vi "User Update Table for Spartan 5.0.vi"(8 "error in (no error)":errorcluster, 11 "Connection Refnum":T1) -> (0 "error out":errorcluster, 3 "Connection Refnum":T1)   [LabVIEW 2011]
uses:
  SI.LIB/ODBC/SQL Controls/Connection Refnum.ctl
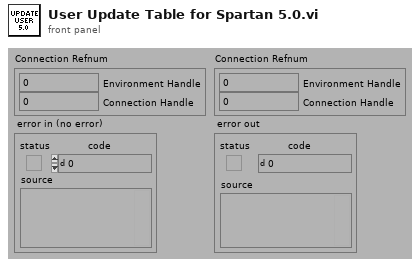
[diagram p1: front panel]
types:
  T1 = typedef "Connection Refnum.ctl" = cluster{"Environment Handle":i32, "Connection Handle":i32}
  T2 = typedef "Statement Refnum.ctl" = cluster{"Statement Handle":i32, "Parameter Number":u16}
  T3 = typedef "User Record.ctl" = cluster{"ixUser":i32, "sxUsername":string, "sLastName":string, "sFirstName":string, "sEmail":string, "sPassword":string, "tLoginTime":timestamp, "sLoginComputer":string, "fAdministrator":bool, "fRunSequences":bool, "fModifySequences":bool, "fRunScenarios":bool, "fModifyScenarios":bool, "fModifyTemplates":bool, "fModifyUsers":bool, "fModifyStations":bool, "fModifyFields":bool}
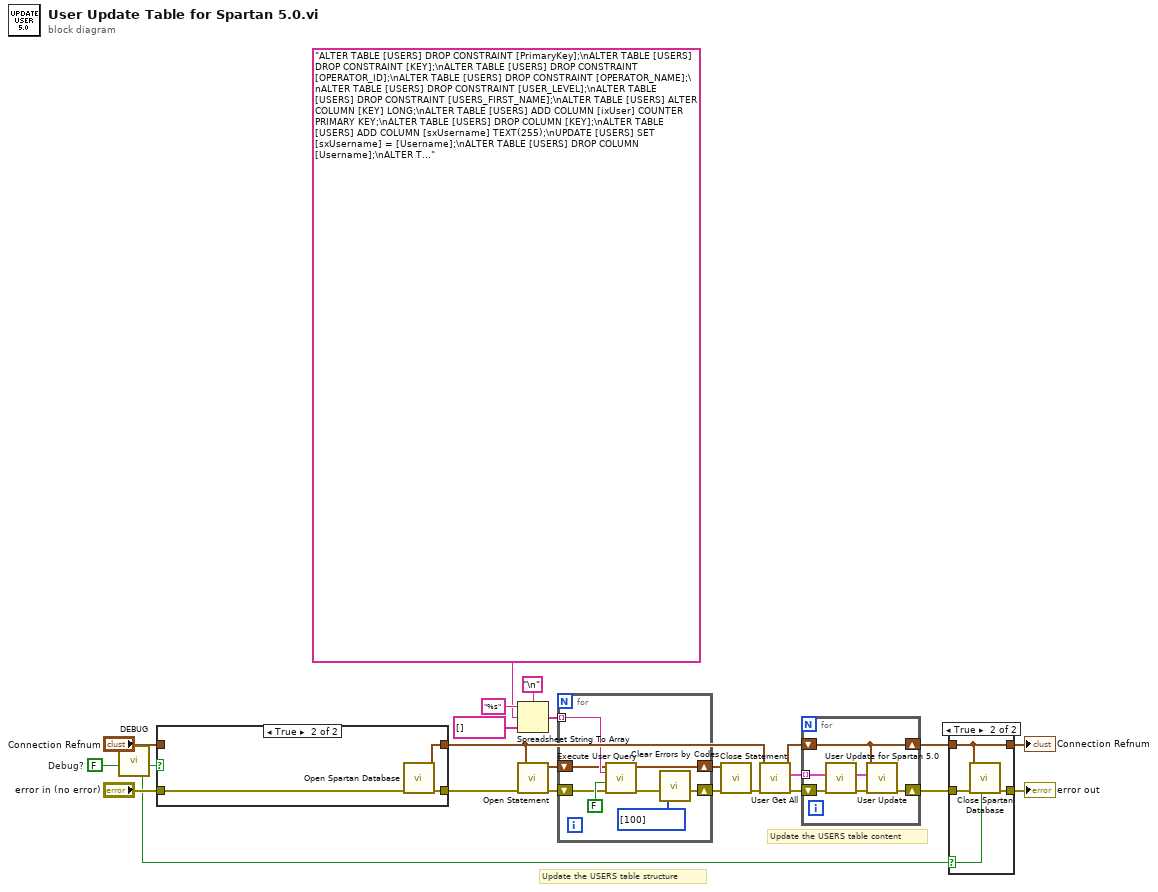
[diagram p0: block diagram]
diagram:
  w10 = FALSE  # Debug?
  # "Update the USERS table content"
  # "Update the USERS table structure"
  n1 = call "DEBUG.vi"("Dev DEBUG? (f)"=w10) -> ("DEBUG?"=w9:bool)  [unwired: 1 in, 5 out]
  n2 = case shown="True" w9 {
    tunnel: "Connection Refnum" -> [w25 _]
    tunnel: "error in (no error)" -> [w24 w28]
    tunnel: [w24 w27] -> w11
    tunnel: [w25 w26] -> w5
    frame False {
    }
    frame True {
      n3 = call "Open Spartan Database.vi"("error in (no error)"=w28) -> ("error out"=w27:errorcluster, "Connection Refnum"=w26:T1)  [unwired: 2 in, 7 out]
    }
  }
  n4 = Spreadsheet String To Array(delimiter (Tab)="\n", format string="%s", spreadsheet string="ALTER TABLE [USERS] DROP CONSTRAINT [PrimaryKey];\nALTER TABLE [USERS] DROP CONSTRAINT [KEY];\nALTER TABLE [USERS] DROP CONSTRAINT [OPERATOR_ID];\nALTER TABLE [USERS] DROP CONSTRAINT [OPERATOR_NAME];\nALTER TABLE [USERS] DROP CONSTRAINT [USER_LEVEL];\nALTER TABLE [USERS] DROP CONSTRAINT [USERS_FIRST_NAME];\nALTER TABLE [USERS] ALTER COLUMN [KEY] LONG;\nALTER TABLE [USERS] ADD COLUMN [ixUser] COUNTER PRIMARY KEY;\nALTER TABLE [USERS] DROP COLUMN [KEY];\nALTER TABLE [USERS] ADD COLUMN [sxUsername] TEXT(255);\nUPDATE [USERS] SET [sxUsername] = [Username];\nALTER TABLE [USERS] DROP COLUMN [Username];\nALTER TABLE [USERS] ADD COLUMN [sLastName] TEXT(255);\nUPDATE [USERS] SET [sLastName] = [Last_Name];\nALTER TABLE [USERS] DROP COLUMN [Last_Name];\nALTER TABLE [USERS] ADD COLUMN [sFirstName] TEXT(255);\nUPDATE [USERS] SET [sFirstName] = [First_Name];\nALTER TABLE [USERS] DROP COLUMN [First_Name];\nALTER TABLE [USERS] ADD COLUMN [sEmail] TEXT(255);\nUPDATE [USERS] SET [sEmail] = [Email];\nALTER TABLE [USERS] DROP COLUMN [Email];\nALTER TABLE [USERS] ADD COLUMN [sPassword] TEXT(255);\nUPDATE [USERS] SET [sPassword] = [Passhash];\nALTER TABLE [USERS] DROP COLUMN [Passhash];\nALTER TABLE [USERS] ADD COLUMN [tLoginTime] DATE;\nALTER TABLE [USERS] ADD COLUMN [sTemp1] TEXT(255);\nUPDATE [USERS] SET [sTemp1] = [Login_Time];\nALTER TABLE [USERS] DROP COLUMN [Login_Time];\nALTER TABLE [USERS] ADD COLUMN [sLoginComputer] TEXT(255);\nUPDATE [USERS] SET [sLoginComputer] = [Login_Computer];\nALTER TABLE [USERS] DROP COLUMN [Login_Computer];\nALTER TABLE [USERS] ADD COLUMN [fAdministrator] LONG;\nALTER TABLE [USERS] ADD COLUMN [fRunSequences] LONG;\nALTER TABLE [USERS] ADD COLUMN [fModifySequences] LONG;\nALTER TABLE [USERS] ADD COLUMN [fRunScenarios] LONG;\nALTER TABLE [USERS] ADD COLUMN [fModifyScenarios] LONG;\nALTER TABLE [USERS] ADD COLUMN [fModifyTemplates] LONG;\nALTER TABLE [USERS] ADD COLUMN [fModifyUsers] LONG;\nALTER TABLE [USERS] ADD COLUMN [fModifyStations] LONG;\nALTER TABLE [USERS] ADD COLUMN [fModifyFields] LONG;\nALTER TABLE [USERS] ADD COLUMN [sTemp2] TEXT(255);\nUPDATE [USERS] SET [sTemp2] = [Permissions];\nALTER TABLE [USERS] DROP COLUMN [Permissions];\nUPDATE [USERS] SET [sPassword] = [sPassword]+'-'+[sTemp1]+'-'+[sTemp2];\nALTER TABLE [USERS] DROP COLUMN [sTemp1];\nALTER TABLE [USERS] DROP COLUMN [sTemp2];\nALTER TABLE [USERS] DROP COLUMN [User_Level];" ("User Query"), array type (2D Dbl)=string[] []) -> (array=w22:string[])
  n5 = call "Open Statement.vi"("error in (no error)"=w11, "Connection Refnum"=w5) -> ("error out"=w19:errorcluster, "Statement Refnum"=w18:T2)  [unwired: 4 out]
  n6 = for {
    shift-right: [w29] -> w17
    shift-left: w19 -> [w33]
    tunnel: w22 -> [w35] mode=indexing
    shift-right: [w32] -> w16
    shift-left: w18 -> [w34]
    n7 = call "Execute User Query.vi"("error in (no error)"=w33, "Return Data? (f)"=FALSE, "User Query"=w35, "Statement Refnum"=w34) -> ("error out"=w30:errorcluster, "Statement Refnum"=w32:T2)  [unwired: 2 out]
    n8 = call "Clear Errors by Codes.vi"("Error Codes\nto Clear (Empty)"=i32[] [100] ("Error Codes\nto Clear (Empty)"), "error in (no error)"=w30) -> ("error out"=w29:errorcluster)  [unwired: 5 out]
  }
  n9 = call "Close Statement.vi"("error in (no error)"=w17, "Statement Refnum"=w16) -> ("error out"=w4:errorcluster)  [unwired: 5 out]
  n10 = call "User Get All.vi"("error in (no error)"=w4, "Connection Refnum"=w5) -> ("error out"=w6:errorcluster, "User Records"=w8:T3[], "Connection Refnum"=w7:T1)  [unwired: 2 in, 5 out]
  n11 = for {
    shift-right: [w42] -> w3
    shift-left: w6 -> [w40]
    shift-right: [w41] -> w2
    shift-left: w7 -> [w41]
    tunnel: w8 -> [w37] mode=indexing
    n12 = call "User Update for Spartan 5.0.vi"("error in (no error)"=w40, "Old User Record"=w37) -> ("error out"=w39:errorcluster, "New User Record"=w38:T3)  [unwired: 8 out]
    n13 = call "User Update.vi"("error in (no error)"=w39, "User Record"=w38, "Connection Refnum"=w41) -> ("error out"=w42:errorcluster)  [unwired: 8 out]
  }
  n14 = case shown="True" w9 {
    selector: w9 -> [_ w46]
    tunnel: w3 -> [w44 w48]
    tunnel: w2 -> [w43 w45]
    tunnel: [w43 w45] -> w15
    tunnel: [w44 w47] -> w14
    frame False {
    }
    frame True {
      n15 = call "Close Spartan Database.vi"("Force Close? (f)"=w46, "error in (no error)"=w48, "Connection Refnum"=w45) -> ("error out"=w47:errorcluster)  [unwired: 2 in, 6 out]
    }
  }
  "error out" <- w14
  "Connection Refnum" <- w15
